vi "tester.vi"() -> ()   [LabVIEW 2016]
uses:
  <vilib>/NI/JSON Support for LabVIEW/JSON Data Classes/JSON Array/JSON Array.lvclass
  C:/Program Files (x86)/National Instruments/LabVIEW 2016/vi.lib/NI/JSON Support for LabVIEW/JSON Data Classes/JSON Datatype/JSON Null.lvclass
  <vilib>/NI/JSON Support for LabVIEW/JSON Data Classes/JSON Array/New JSON Array (Numeric).vi
  <vilib>/NI/NI JSONRPC Server Framework/Classes/Server/Format Client Request (Auto-Increment).vi
  <vilib>/httpClient/POSTBuffer.vi
  <vilib>/NI/NI JSONRPC Server Framework/Classes/Server/JSONRPC Server.lvclass
  <vilib>/NI/JSON Support for LabVIEW/JSON Data Classes/JSON Helper/JSON Helper.lvclass
  <vilib>/httpClient/LabVIEWHTTPClient.lvlib
  C:/Program Files (x86)/National Instruments/LabVIEW 2016/vi.lib/NI/JSON Support for LabVIEW/JSON Data Classes/JSON Structured Type/JSON Structure.lvclass
panel:
  out "body":string
  in  "second":dbl
  in  "first":dbl
  in  "method":string
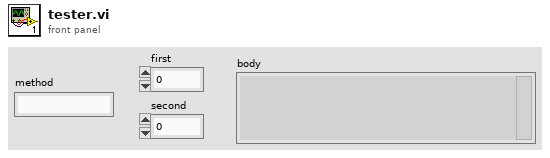
[diagram p1: front panel]
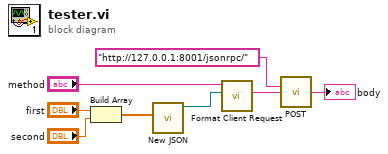
[diagram p0: block diagram]
diagram:
  n1 = Build Array("first", "second") -> (w5:dbl[])
  n2 = call-poly <vilib>:"New JSON.vi"("Numeric Array"=w5) -> ("JSON Array out"=w4:refnum<class "JSON Array.lvclass">)  [unwired: 9 in, 1 out]
  n3 = call-poly <vilib>:"Format Client Request.vi"("JSON in"=w4, "method"="method") -> ("Request String"=w2:string)  [unwired: 8 in, 1 out]
  n4 = call-poly <vilib>:"POST.vi"("url"="http://127.0.0.1:8001/jsonrpc/", "buffer"=w2) -> ("body"=→"body":string)  [unwired: 10 in, 3 out]
